vi "Send Message.vi"(6 "Name":string, 7 "Priority (normal)":T1, 8 "error in (no error)":errorcluster, 10 "Payload":variant, 11 "Actor API in":refnum<class "Actor API.lvclass">) -> (0 "error out":errorcluster)   [LabVIEW 2020, in "Actor API.lvclass"]
uses:
  Actor API.lvclass
  <vilib>/event_ctls.llb/usereventprio.ctl
  Actor/Message.ctl
  Actor API.lvclass/Actor API.ctl
  Actor/Actor.lvclass
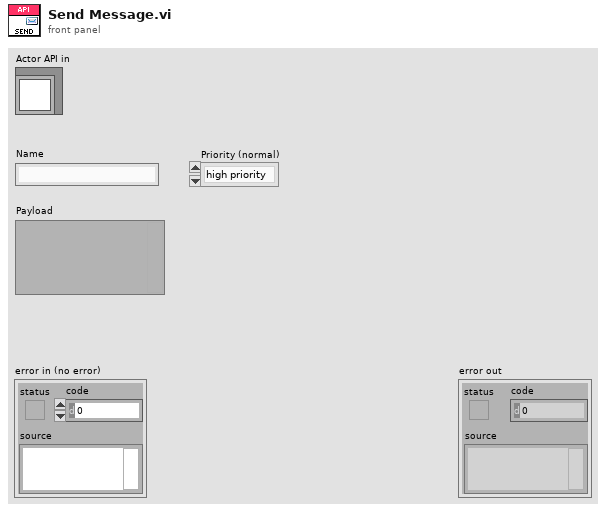
[diagram p1: front panel]
types:
  T1 = typedef "usereventprio.ctl" = enum32{"high priority", "normal priority"}
  T2 = typedef "Actor.lvclass/Message.ctl" = cluster{"Name":string, "Payload":variant}
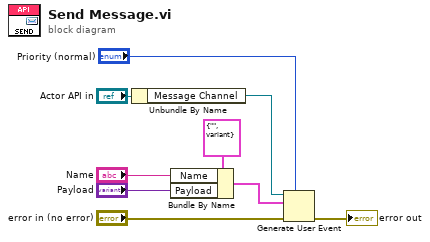
[diagram p0: block diagram]
diagram:
  n1 = Unbundle By Name("Actor API in") -> ("Message Channel"=w6:refnum<user-event>)
  n2 = Bundle By Name(cluster=T2 {"Name"="", "Payload"=variant} ("Message"), "Name"="Name", "Payload"="Payload") -> (w2:T2)
  n3 = Generate User Event(priority (normal)="Priority (normal)", user event=w6, event data cluster=w2, error in="error in (no error)") -> (error out=→"error out":errorcluster)  [unwired: 1 out]
